vi "Voltage - Continuous Input-ExtClk.vi"() -> ()   [LabVIEW 2014]
doc: "This example demonstrates how to acquire a single buffer of voltage measurements using a DAQmx device.\n\nFor instructions on how to connect your signals to the DAQ device, refer to your device documentation."
uses:
  <vilib>/Utility/error.llb/DialogType.ctl
  <vilib>/DAQmx/create/channels.llb/DAQmx Create Channel (AI-Voltage-Basic).vi
  <vilib>/DAQmx/configure/timing.llb/DAQmx Timing (Sample Clock).vi
  <vilib>/DAQmx/read.llb/DAQmx Read (Analog Wfm 1Chan NSamp).vi
panel:
  in  "Stop":bool
  out "Waveform Graph":waveform(dbl)(graph)
  in  "Number of Samples":i32=100
  in  "Sample Rate":dbl=1000.0
  in  "Sample Clock Source":tag="PFI0"
  in  "Terminal Configuration":i32(ring)=-1 items=["default"=-1, "RSE"=10083, "NRSE"=10078, "Differential"=10106, "Pseudodifferential"=12529]
  in  "Max Voltage":dbl=5.0
  in  "Min Voltage":dbl=-5.0
  in  "Physical Channel":tag="Dev1/ai0"
  # "Channel Settings"
  # "Acquired Data"
  # "Timing Settings"
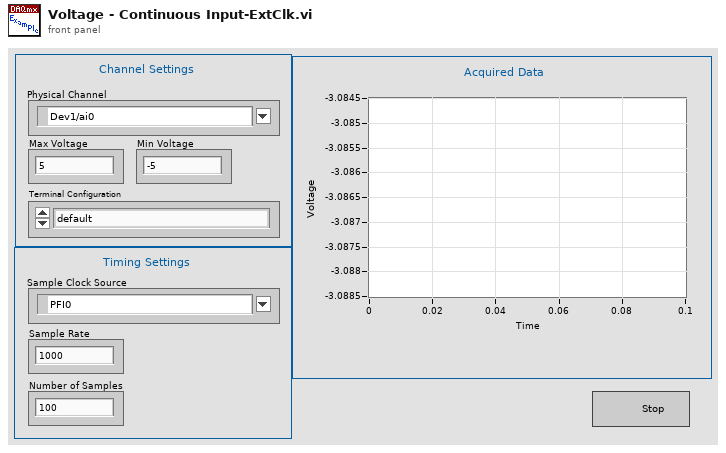
[diagram p1: front panel]
types:
  T1 = typedef "DialogType.ctl" = u16
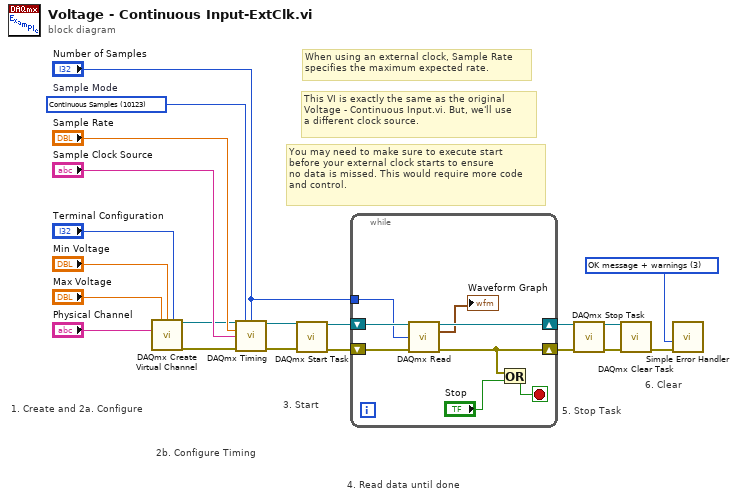
[diagram p0: block diagram]
diagram:
  w5 = T1 3 items=["no dialog", "OK message", "continue or stop message", "OK message + warnings", "continue/stop + warnings"] ("type of dialog (OK msg:1)")
  w20 = 10123 items=["Finite Samples"=10178, "Continuous Samples"=10123, "Hardware Timed Single Point"=12522]  # Sample Mode
  # "You may need to make sure to execute start \nbefore your external clock starts to ensure\nno data is missed. This would require more code\nand control."
  # "When using an external clock, Sample Rate\nspecifies the maximum expected rate."
  # "This VI is exactly the same as the original\nVoltage - Continuous Input.vi. But, we'll use\na different clock source."
  # "2b. Configure Timing"
  # "6. Clear"
  # "5. Stop Task"
  # "3. Start"
  # "4. Read data until done"
  # "1. Create and 2a. Configure"
  n1 = call-poly <vilib>:"DAQmx Create Virtual Channel.vi"("maximum value"="Max Voltage", "minimum value"="Min Voltage", "input terminal configuration"="Terminal Configuration", "physical channels"="Physical Channel") -> ("task out"=w4:refnum<k21>, "error out"=w19:errorcluster)  [unwired: 10 in]
  n2 = call-poly <vilib>:"DAQmx Timing.vi"("task/channels in"=w4, "sample mode"=w20, "samples per channel"="Number of Samples", "rate"="Sample Rate", "source"="Sample Clock Source", "error in"=w19) -> ("task out"=w3:refnum<k21>, "error out"=w2:errorcluster)  [unwired: 8 in]
  n3 = call <vilib>:"DAQmx Start Task.vi"("task/channels in"=w3, "error in"=w2) -> ("task out"=w18:refnum<k21>, "error out"=w17:errorcluster)  [unwired: 12 in]
  n4 = while {
    shift-right: [w26] -> w7
    shift-left: w18 -> [w28]
    shift-right: [w24] -> w6
    shift-left: w17 -> [w27]
    tunnel: "Number of Samples" -> [w22]
    stop <- w25 stop-if-true
    n5 = call-poly <vilib>:"DAQmx Read.vi"("task/channels in"=w28, "number of samples per channel"=w22, "error in"=w27) -> ("task out"=w26:refnum<k21>, "data"=→"Waveform Graph":waveform(dbl), "error out"=w24:errorcluster)  [unwired: 10 in]
    n6 = Or(x=w24, y="Stop") -> (x .or. y?=w25:bool)
  }
  n7 = call <vilib>:"DAQmx Stop Task.vi"("task/channels in"=w7, "error in"=w6) -> ("task out"=w9:refnum<k21>, "error out"=w8:errorcluster)  [unwired: 12 in]
  n8 = call <vilib>:"DAQmx Clear Task.vi"("task in"=w9, "error in"=w8) -> ("error out"=w16:errorcluster)  [unwired: 13 in]
  n9 = call <vilib>:"Simple Error Handler.vi"("type of dialog (OK msg:1)"=w5, "error in (no error)"=w16) -> ()  [unwired: 3 in, 5 out]
